vi "Send Message.vi"(8 "error in (no error)":errorcluster, 9 "data (JSON)":string, 10 "msg (string)":string, 11 "WebSocket Connection in":refnum<k5>) -> (0 "error out":errorcluster, 3 "WebSocket Connection out":refnum<k5>)   [LabVIEW 2014]
uses:
  <vilib>/Intelligent Energy/WebSockets API/WebSockets/WebSockets.lvlib
panel:
  in  "timeout ms (5000)":i32=5000
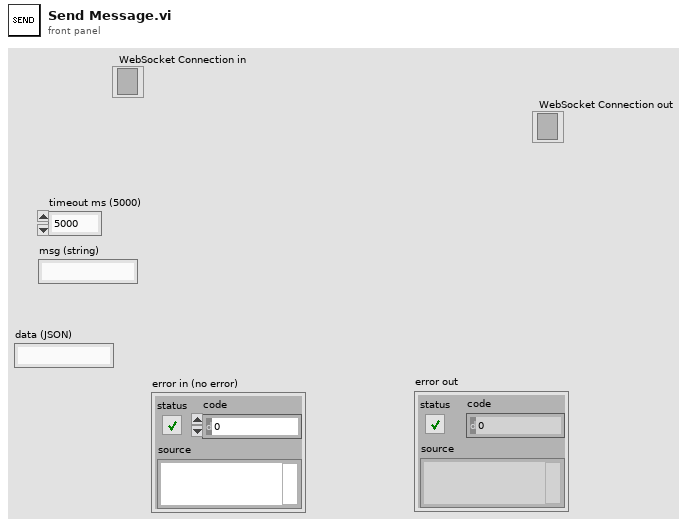
[diagram p1: front panel]
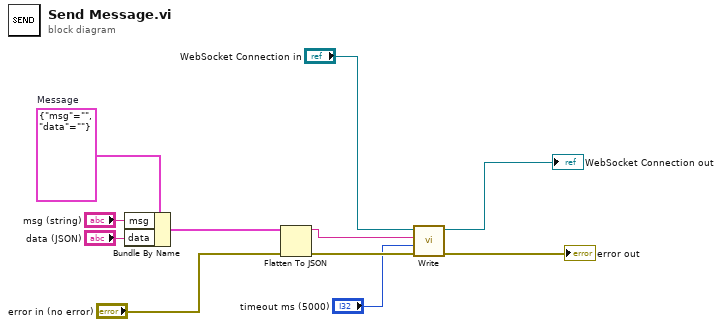
[diagram p0: block diagram]
diagram:
  w9 = cluster{"msg":string, "data":string} {"msg"="", "data"=""}  # Message
  n1 = Bundle By Name(cluster=w9, "msg"="msg (string)", "data"="data (JSON)") -> (w8:cluster{"msg":string, "data":string})
  n2 = Flatten To JSON(anything=w8, error in (no error)="error in (no error)") -> (JSON string=w6:string, 11:w7:errorcluster)  [unwired: 1 in]
  n3 = call <vilib>:"Write.vi"("error in (no error)"=w7, "timeout ms (5000)"="timeout ms (5000)", "Data"=w6, "WebSocket Connection in"="WebSocket Connection in") -> ("error out"=→"error out":errorcluster, "WebSocket Connection out"=→"WebSocket Connection out":refnum<k5>)  [unwired: 6 in]
